vi "uActor_SimpleSend.vi"(5 "Reply CMD (re:<cmd>)":string, 6 "Timestamp (Now)":u32, 7 "Reply Transport":refnum<class "uTransport.lvclass">, 8 "error in (no error)":errorcluster, 9 "Payload":refnum<class "uData.lvclass">, 10 "Msg":string, 11 "uActor Transport":refnum<class "uTransport_uActor.lvclass">) -> (0 "error out":errorcluster)   [LabVIEW 2023, in "uLib.lvlib" / "uActor.lvclass"]
doc: "Simplified method to message the actor. For full control, use the send_message instead.\nThis is inlined to optimize for performance when the class is statically dispatched. For generic calls, the 'uTransport_SimpleSend' may be used.\n\nA blank string is a NULL message whose reponse may NOT be overriden by the children using the EXEC method."
uses:
  uActor.lvclass
  uTransport/uTransport_uActor/uTransport_uActor.lvclass
  uTransport/uTransport/uTransport.lvclass
  uData/uData/uData.lvclass
  uMsg/uMsg/uMsg.lvclass/uMsg.ctl
  uTransport/uTransport_uActor/uTransport_uActor.lvclass/uTransport_uActor.ctl
  uTransport/uTransport_uActor/uTransport_uActor_SendMsg.vi
  uMsg/uMsg/uMsg Update Timestamp.vi
  uMsg/uMsg/uMsg.lvclass
  uActor.lvclass/uActor.ctl
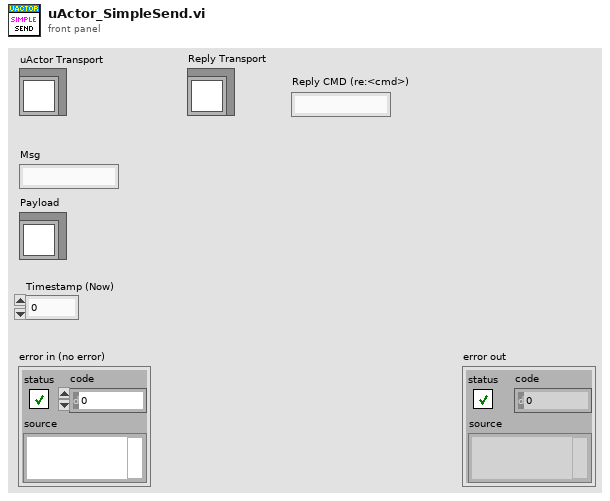
[diagram p1: front panel]
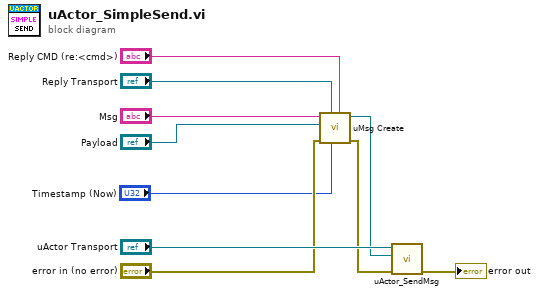
[diagram p0: block diagram]
diagram:
  n1 = call "uMsg Create.vi"("Reply CMD (re:<cmd>)"="Reply CMD (re:<cmd>)", "Timestamp (NULL)"="Timestamp (Now)", "Reply Transport"="Reply Transport", "error in (no error)"="error in (no error)", "Payload"="Payload", "CMD"="Msg") -> ("error out"=w5:errorcluster, "uMsg out"=w4:refnum<class "uMsg.lvclass">)  [unwired: 4 in]
  n2 = call "uActor_SendMsg.vi"("error in (no error)"=w5, "Msg"=w4, "uActor Transport"="uActor Transport") -> ("error out"=→"error out":errorcluster)  [unwired: 8 in]
